vi "COMI ENC Reset.vi"(10 "ch":i32, 11 "hDevice":u32) -> (3 "hDevice out":u32)   [LabVIEW 2017, in "Comidll.lvlib"]
doc: "void (COMI_ENC_Reset) (HANDLE hDevice, int ch);"
uses:
  <userlib>/Comidll/Comidll.lvlib
  <userlib>/Comidll/Comidll.dll
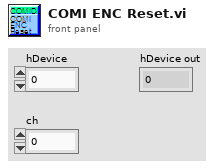
[diagram p1: front panel]
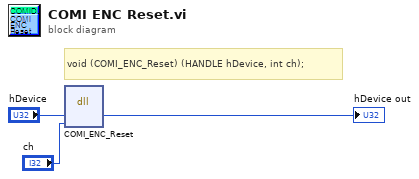
[diagram p0: block diagram]
diagram:
  # "void\t(COMI_ENC_Reset) (HANDLE hDevice, int ch);"
  n1 = dll-call lib="C:/Program Files/National Instruments/LabVIEW 2017/user.lib/Comidll/Comidll.*" fn="COMI_ENC_Reset"("hDevice"="hDevice", "ch"="ch") -> ("hDevice"=→"hDevice out":u32)  [unwired: 5 in, 2 out]
